vi "refgen.vi"(7 "refgen":cluster{"slope":dbl, "period":dbl}, 11 "Qube":refnum<class "Qube.lvclass">) -> (1 "r":dbl, 3 "Qube":refnum<class "Qube.lvclass">)   [LabVIEW 2017, in "Qube.lvclass"]
uses:
  Qube.lvclass
  <vilib>/numeric/Random Number (Range) DBL.vi
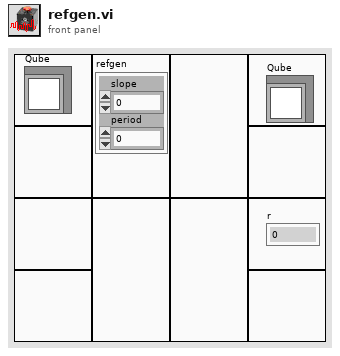
[diagram p1: front panel]
types:
  T1 = typedef "Qube.lvclass/mode.ctl" = enum16{"Control", "Identify"}
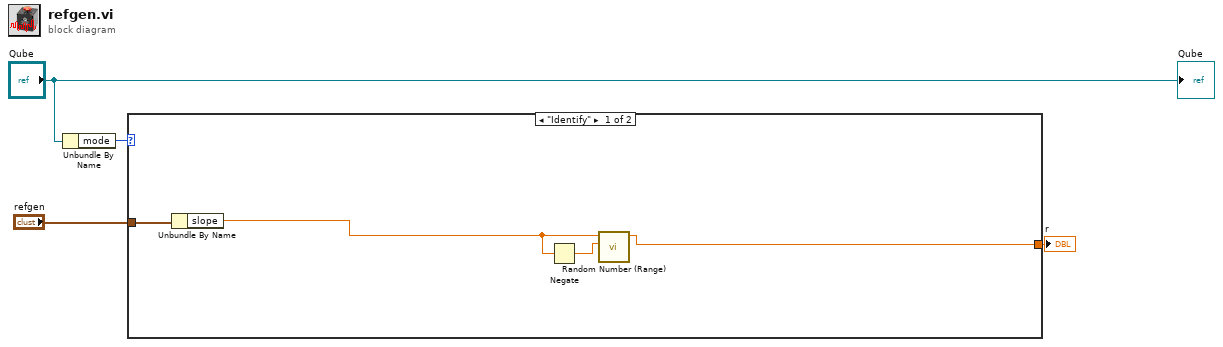
[diagram p0: block diagram]
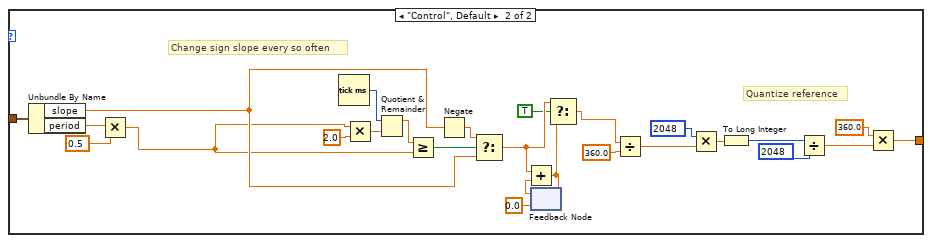
[diagram p2: hidden frame]
diagram:
  n1 = Unbundle By Name("Qube") -> ("mode"=w3:T1)
  n2 = case shown="\"Identify\"" w3 {
    tunnel: [w5 w18] -> w4
    tunnel: "refgen" -> [w8 w34]
    frame "Identify" {
      n3 = Unbundle By Name(w8) -> ("slope"=w6:dbl)
      n4 = Negate(x=w6) -> (-x=w7:dbl)
      n5 = call-poly <vilib>:"Random Number (Range).vi"("lower bound (0)"=w7, "upper bound (100)"=w6) -> ("number"=w5:dbl)  [unwired: 9 in]
    }
    frame "Control", Default {
      # "Change sign slope every so often"
      # "Quantize reference"
      n6 = Unbundle By Name(w34) -> ("slope"=w27:dbl, "period"=w17:dbl)
      n7 = Multiply(x=w17, y=0.5) -> (x*y=w13:dbl)
      n8 = Tick Count (ms)() -> (millisecond timer value=w33:u32)
      n9 = Multiply(x=w13, y=2.0) -> (x*y=w32:dbl)
      n10 = Quotient & Remainder(x=w33, y=w32) -> (x-y*floor(x/y)=w30:dbl)  [unwired: 1 out]
      n11 = Greater Or Equal?(x=w30, y=w13) -> (x >= y?=w29:bool)
      n12 = Negate(x=w27) -> (-x=w28:dbl)
      n13 = Select(t=w28, s=w29, f=w27) -> (s? t:f=w10:dbl)
      n14 = feedback #1(0.0) -> (w15:dbl)
      n15 = Add(x=w10, y=w15) -> (x+y=w11:dbl)
      n16 = feedback-in #1(w11) -> ()
      n17 = Select(t=w10, s=TRUE, f=w11) -> (s? t:f=w12:dbl)
      n18 = Divide(x=w12, y=360.0) -> (x/y=w24:dbl)
      n19 = Multiply(x=2048 ("y"), y=w24) -> (x*y=w25:dbl)
      n20 = To Long Integer(number=w25) -> (32bit integer=w26:i32)
      n21 = Divide(x=w26, y=2048) -> (x/y=w23:dbl)
      n22 = Multiply(x=360.0, y=w23) -> (x*y=w18:dbl)
    }
  }
  "r" <- w4
  "Qube" <- "Qube"
